vi "Spec Limit Line.vi"(8 "Index":i32, 9 "Spec Association Col No":string[](array[string])=["1", "2", "3", "4", "NAN", "NAN", "NAN", "NAN"], 10 "Spec _Data":dbl[][](array[numeric]), 11 "Frequency(Hz)":dbl[](array[numeric])) -> (1 "Spec Number":dbl, 2 "Not NAN":bool, 3 "Limit Spec  Data":T1)   [LabVIEW 2011]
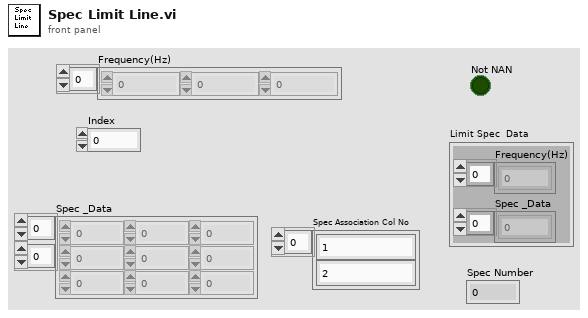
[diagram p1: front panel]
types:
  T1 = cluster{"Frequency(Hz)":dbl[], "Spec _Data":dbl[]}
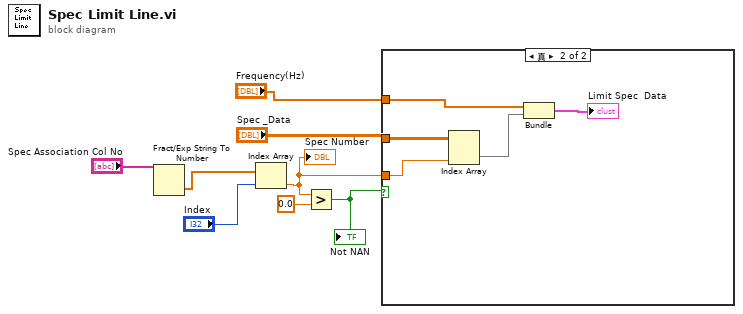
[diagram p0: block diagram]
diagram:
  n1 = Fract/Exp String To Number(string="Spec Association Col No") -> (number=w7:dbl[])  [unwired: 3 in, 1 out]
  n2 = Index Array(array=w7, index="Index") -> (element=w3:dbl)
  "Spec Number" <- w3
  n3 = Greater?(x=w3, y=0.0) -> (0:w1:bool)
  "Not NAN" <- w1
  n4 = case shown="真" w1 {
    tunnel: "Spec _Data" -> [_ w13]
    tunnel: w3 -> [_ w12]
    tunnel: "Frequency(Hz)" -> [_ w11]
    frame False {
    }
    frame True {
      n5 = Index Array(array=w13, index (col)=w12) -> (element=w10:dbl[])  [unwired: 1 in]
      n6 = Bundle("Frequency(Hz)"=w11, "Spec _Data"=w10) -> (→"Limit Spec  Data":T1)  [unwired: 1 in]
    }
  }
